vi "HEWH Draw Until.vi"(7 "error in (no error)":errorcluster) -> (0 "error out":errorcluster, 3 "Condition Cluster Output":T4)   [LabVIEW 2019]
uses:
  Utility/Custom Pallet Controls/Custom Pallet DBL.ctl
  Type Definitions/HEWH Power Elements.ctl
  Utility/Custom Pallet Controls/Custom Pallet Forward.ctl
  Utility/Custom Pallet Controls/Custom Pallet Reverse.ctl
  Type Definitions/HEWH Termination Condition Cluster.ctl
panel:
  in  "Mean Tank Temperature Bool":bool
  in  "Mean Tank Temperature":T1 format="%.2f"
  in  "Time":bool
  in  "RTD Temp":bool
  in  "RTD Decrease":bool
  in  "RTD Out Temperature":T1 format="%.2f"
  in  "Time (Seconds)":T1 format="%.2f"
  in  "Return":T2
  in  "Complete":T3
  in  "Decrease RTD Output\nTemperature By\n(Degrees F)":T1 format="%.2f"
  out "Description":string="Draw Until?"
  in  "Tab Control":enum32{"Page 1", "Page 2"}(tab)
  in  "Condition Cluster Input":T4
  in  "Start Draw":bool
  in  "Power Elements":T5
  # "AND/OR"
  # "Select ONLY complete to draw until any heat source"
  # "Select Only One Condition"
  # "Just Draw Water!"
  # "Condition #1"
  # "Draw Until Any Heat Source"
  # "Condition #2"
  # "Start Dispense Pattern"
  # "Draw Until Specific Heat Source"
  # "Condition #3"
  # "Dispense PRAT Sequence"
  # "Not Working"
  # "Condition #4"
  # "Condition #5"
  # "Condition #6"
  # "Select Only One Condition"
  # "Just Draw Water!"
  # "Condition #1"
  # "Draw Until Any Heat Source"
  # "Condition #2"
  # "Start Dispense Pattern"
  # "Draw Until Specific Heat Source"
  # "Condition #3"
  # "Dispense PRAT Sequence"
  # "Not Working"
  # "Condition #4"
  # "Condition #5"
  # "Condition #6"
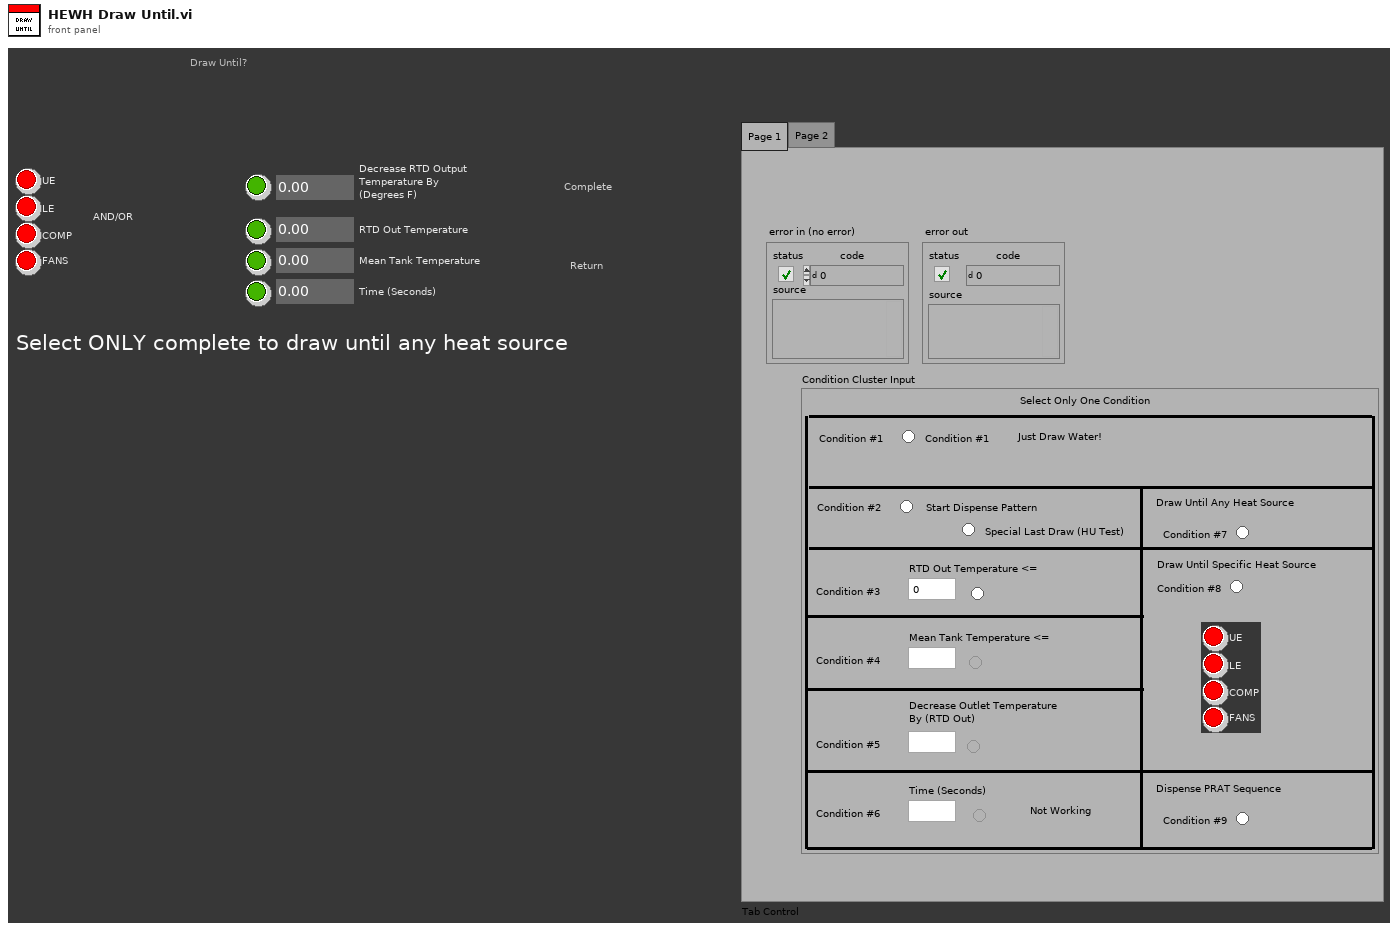
[diagram p1: front panel]
types:
  T1 = typedef "Custom Pallet DBL.ctl" = dbl
  T2 = typedef "Custom Pallet Reverse.ctl" = bool
  T3 = typedef "Custom Pallet Forward.ctl" = bool
  T4 = typedef "HEWH Termination Condition Cluster.ctl" = cluster{"Condition #1":bool, "Condition #2":bool, "Special Last Draw (HU Test)":bool, "RTD Out Temperature <=":dbl, "Condition #3":bool, "Mean Tank Temperature <=":dbl, "Condition #4":bool, "Decrease Outlet Temperature \nBy (RTD Out)":dbl, "Condition #5":bool, "Condition #6":bool, "Time (Seconds)":dbl, "Condition #7":bool, "Condition #8":bool, "Draw Until Condition":T5, "Condition #9":bool}
  T5 = typedef "HEWH Power Elements.ctl" = cluster{"UE":bool, "LE":bool, "COMP":bool, "FANS":bool}
  T6 = enum32{"invalid app kind", "Development System", "Run Time System", "Student Edition", "Embedded LabVIEW", "Evaluation", "Custom"}
  T7 = enum32{"Invalid", "Standard", "Closed", "Hidden", "Minimized", "Maximized"}
  T8 = cluster{"Core":cluster{"Current VI Reference":refnum<vi>, "Close Panel on Exit?":bool}, "Power Elements":T5, "Start Draw":bool, "Decrease RTD Output\nTemperature By\n(Degrees F)":T1, "Return":bool, "Time (Seconds)":T1, "RTD Out Temperature":T1, "Condition Cluster Input":T4, "Mean Tank Temperature":T1}
  T9 = cluster{"Current VI Reference":refnum<vi>, "Close Panel on Exit?":bool}
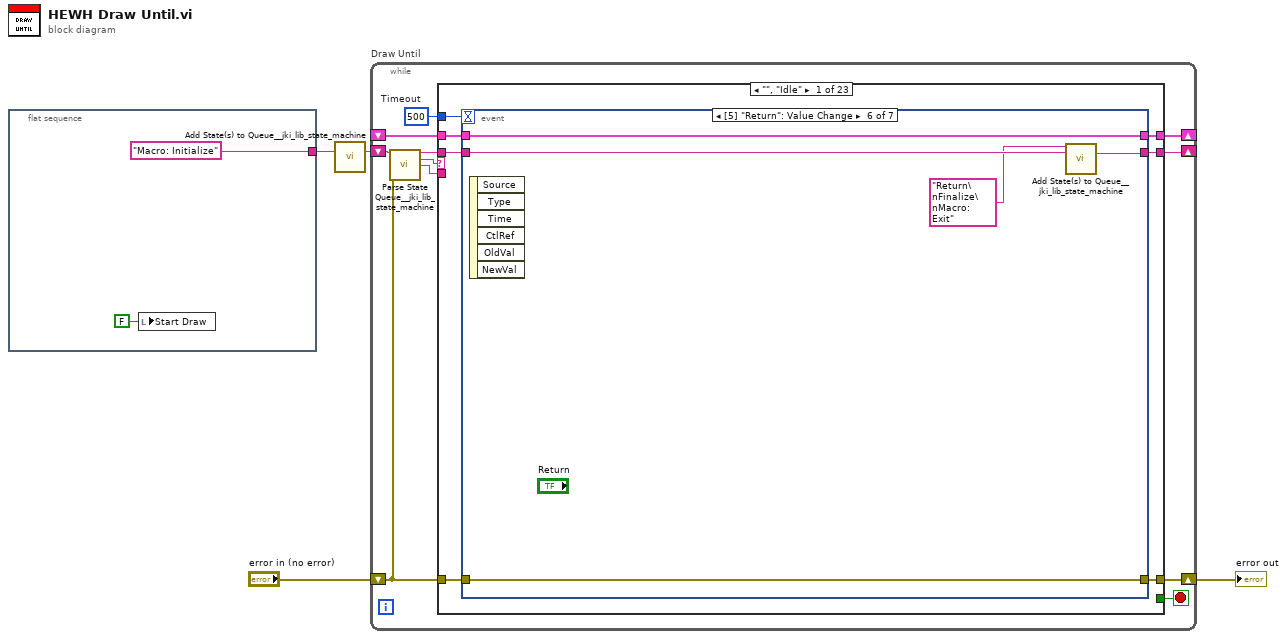
[diagram p0: block diagram]
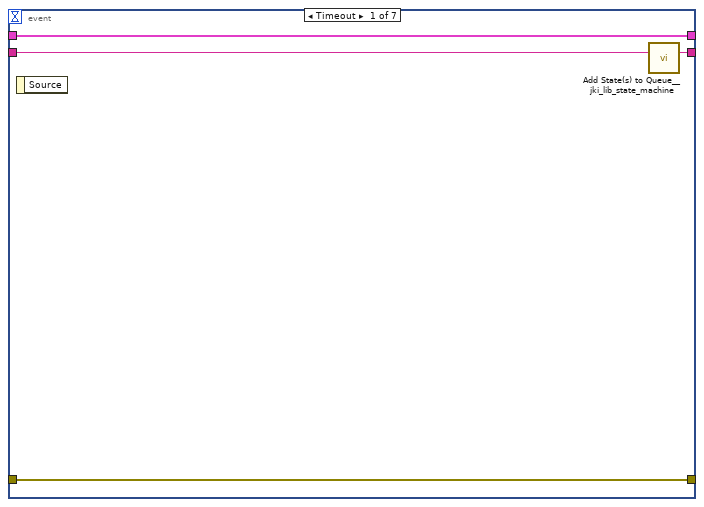
[diagram p2: hidden frame]
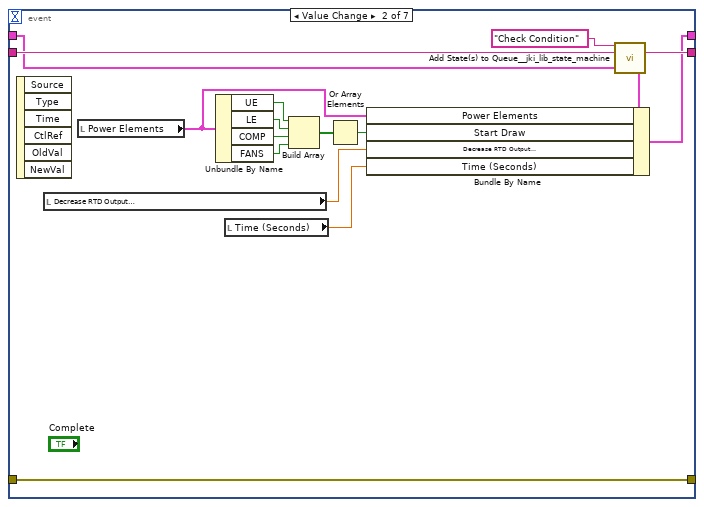
[diagram p3: hidden frame]
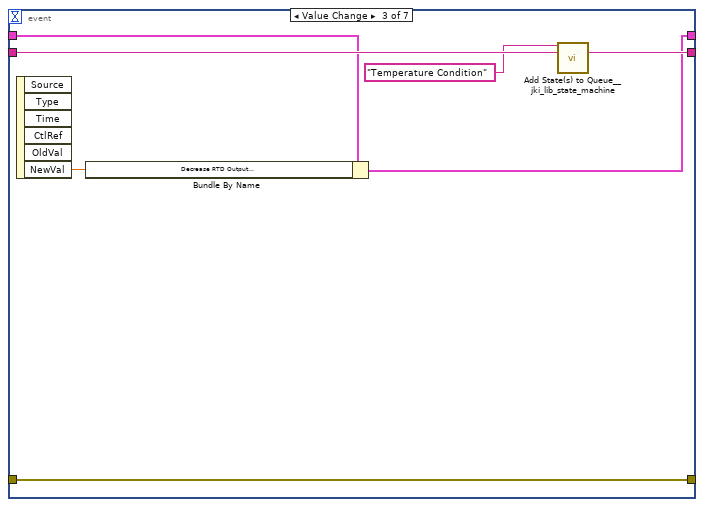
[diagram p4: hidden frame]
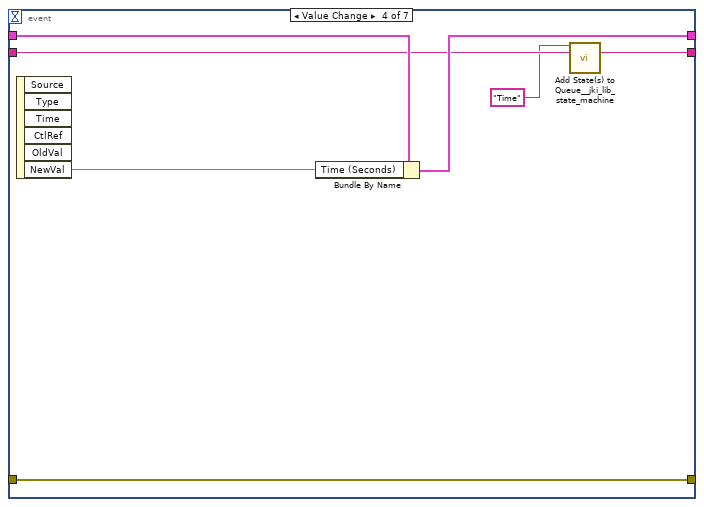
[diagram p5: hidden frame]
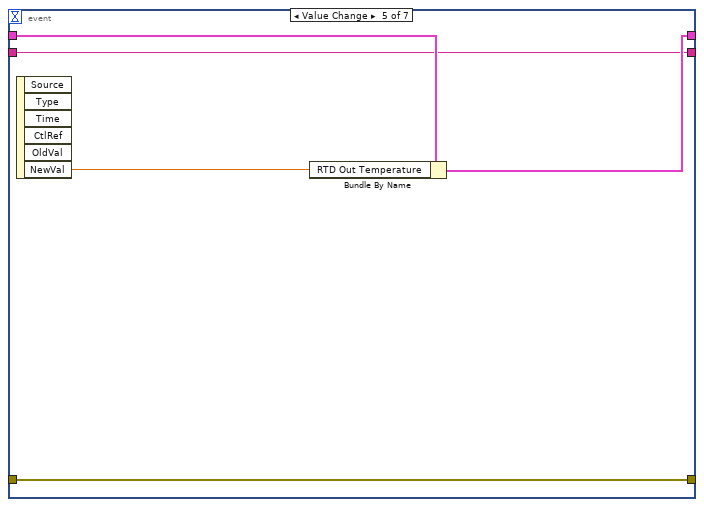
[diagram p6: hidden frame]
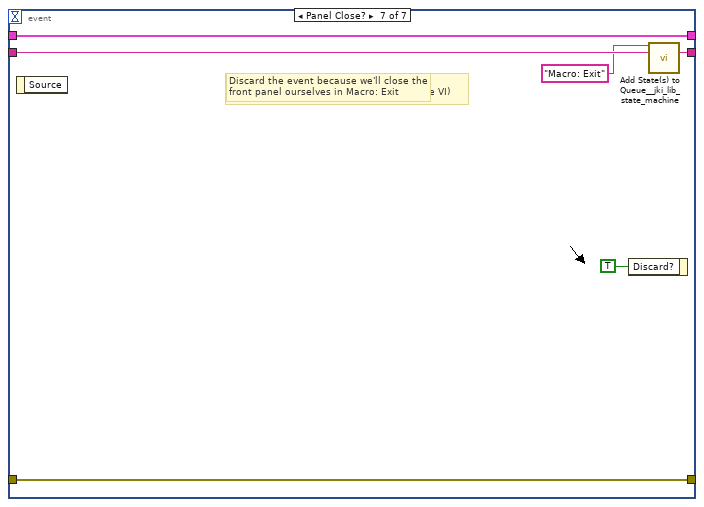
[diagram p7: hidden frame]
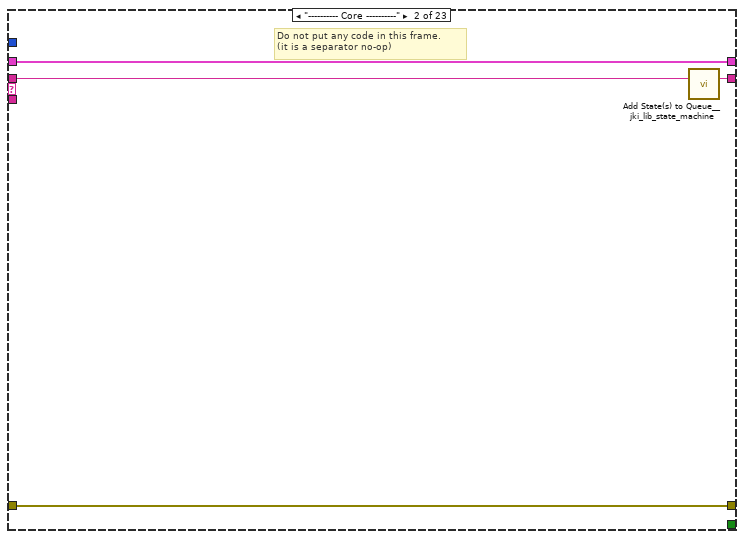
[diagram p8: hidden frame]
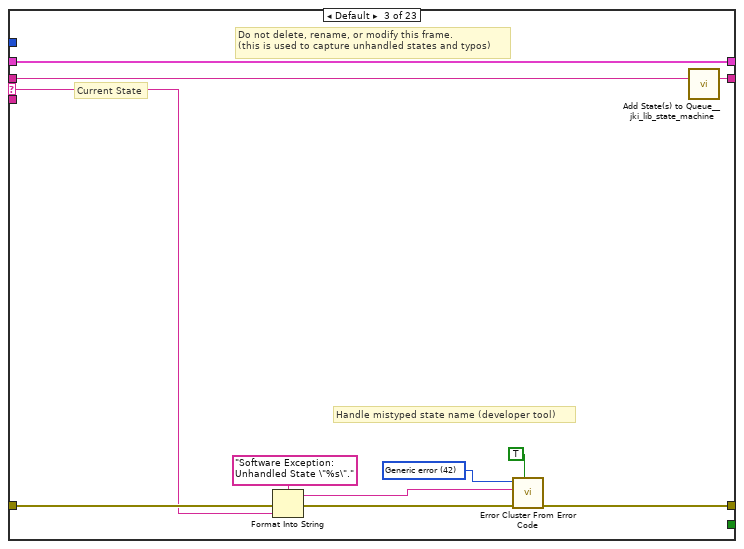
[diagram p9: hidden frame]
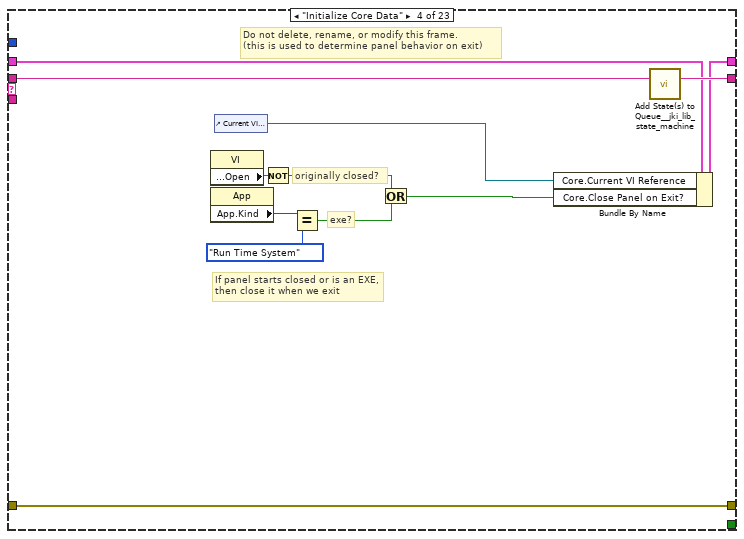
[diagram p10: hidden frame]
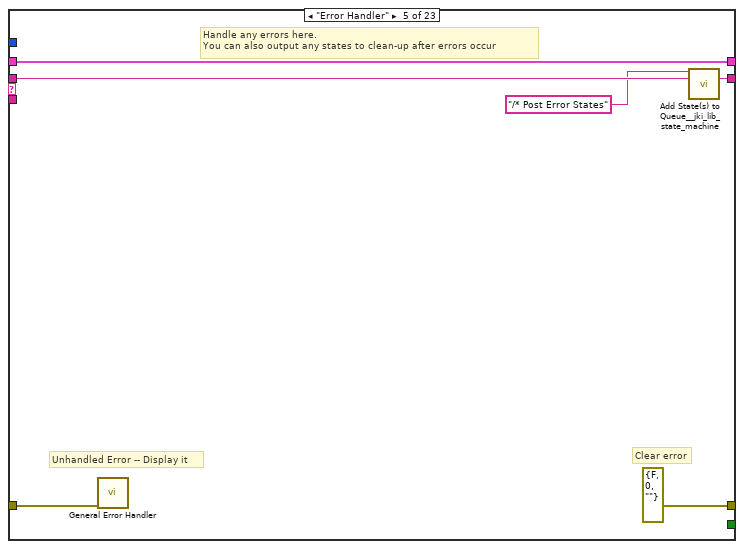
[diagram p11: hidden frame]
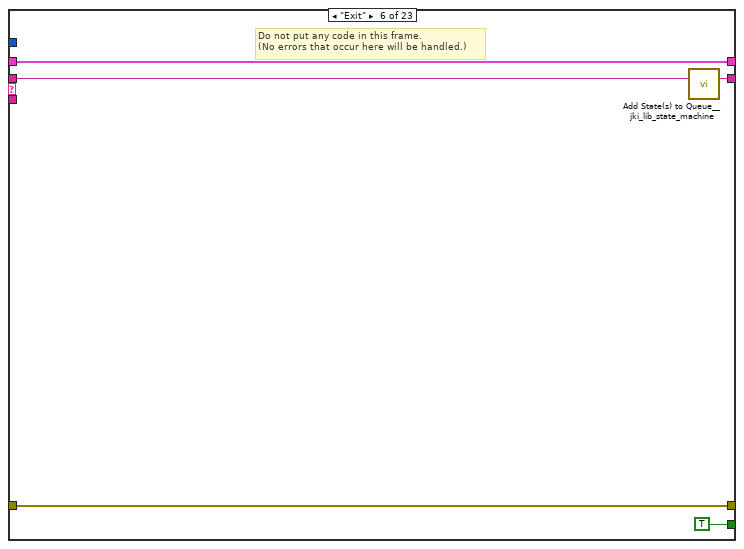
[diagram p12: hidden frame]
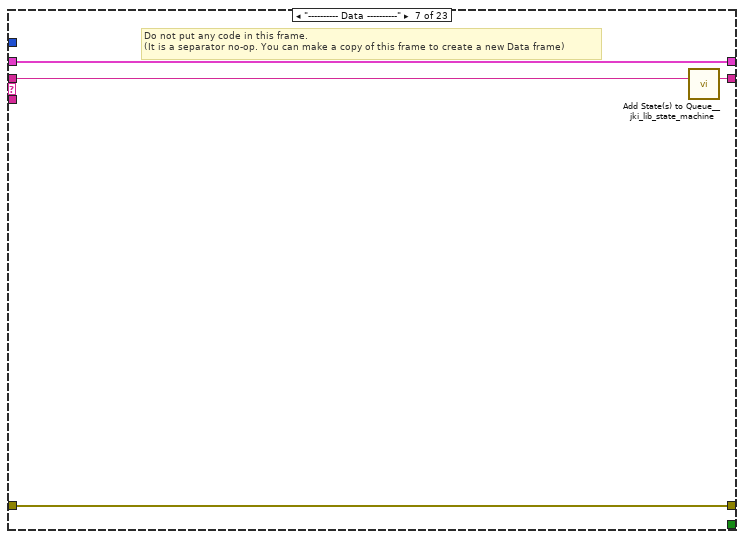
[diagram p13: hidden frame]
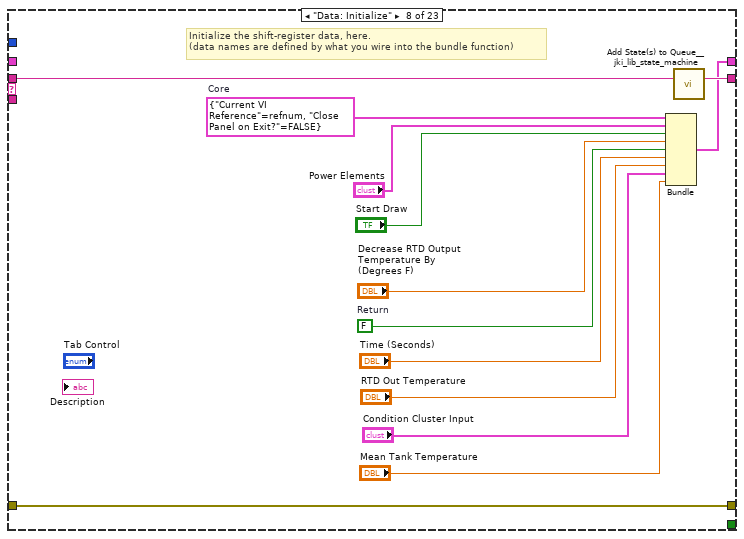
[diagram p14: hidden frame]
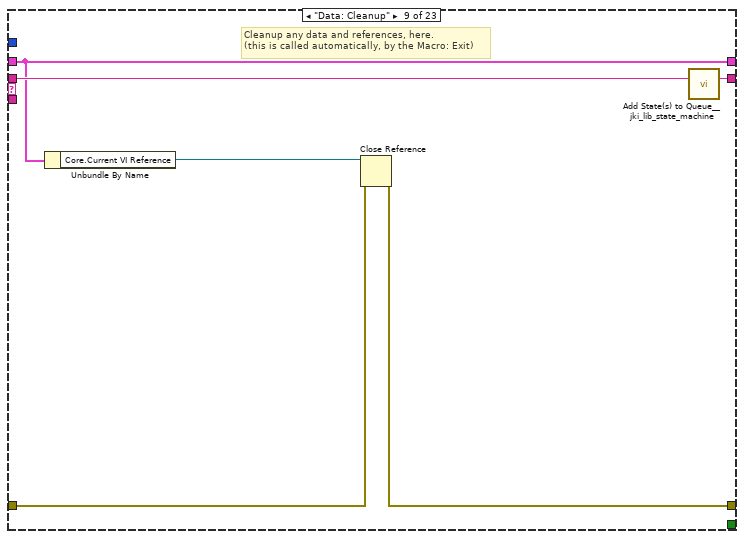
[diagram p15: hidden frame]
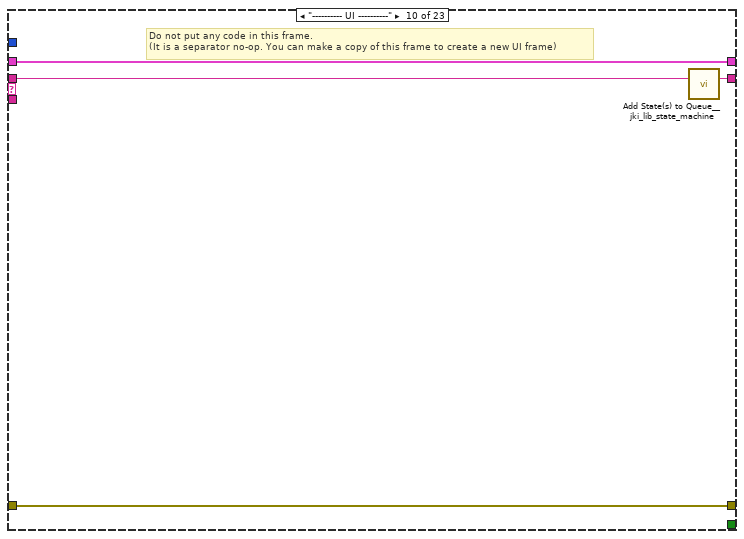
[diagram p16: hidden frame]
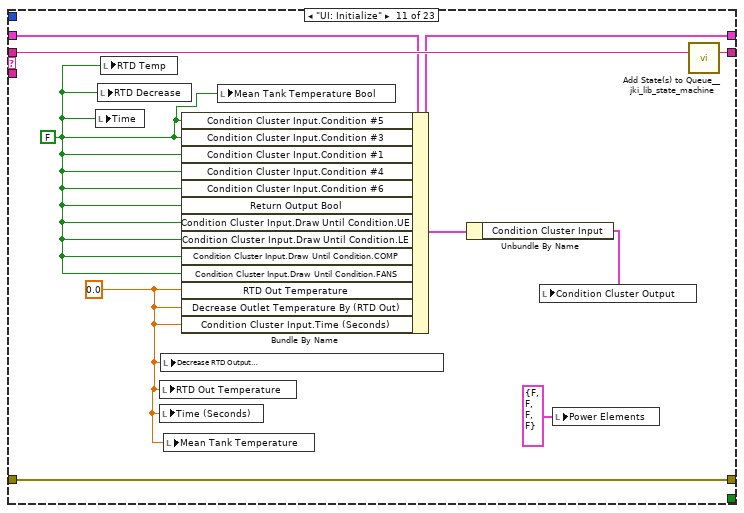
[diagram p17: hidden frame]
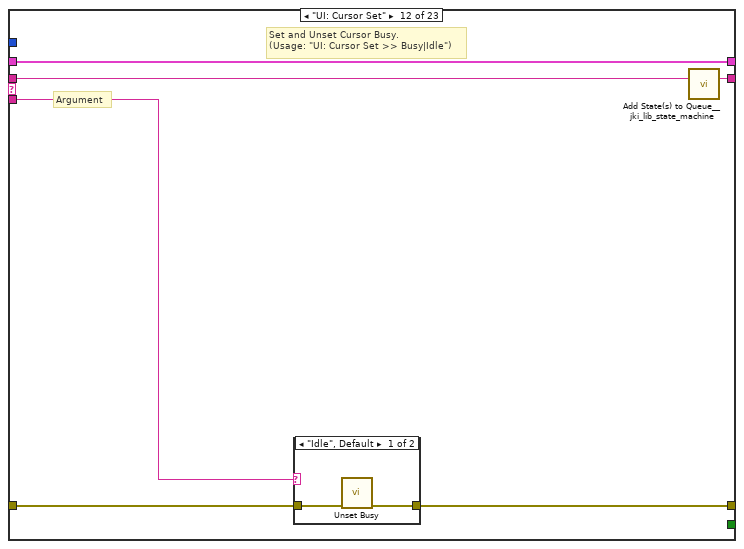
[diagram p18: hidden frame]
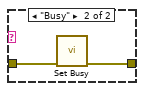
[diagram p19: hidden frame]
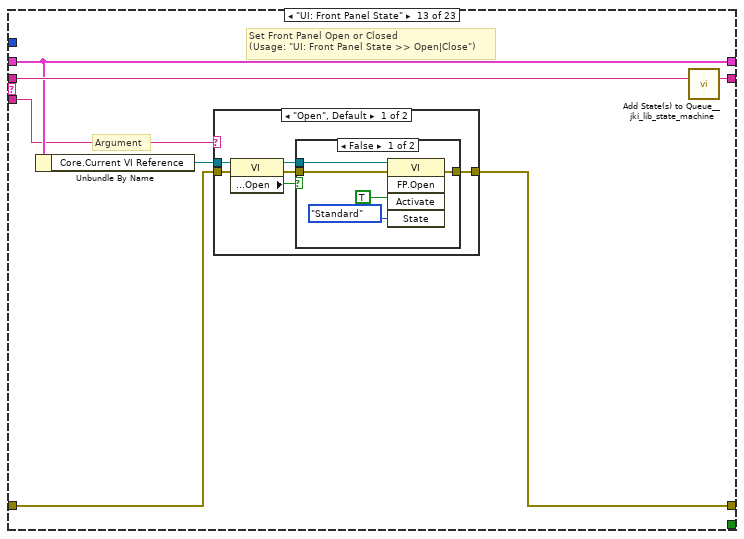
[diagram p20: hidden frame]
diagram:
  n1 = flat-sequence {
    tunnel: ["Macro: Initialize"] -> w3
    frame #0 {
      n2 = local write "Start Draw"(FALSE ("Start Draw")) -> ()
    }
  }
  n3 = call <vilib>:"Add State(s) to Queue__jki_lib_state_machine.vi"("State(s) in (\"\")"=w3) -> ("States Out"=w4:string)  [unwired: 14 in]
  n4 = while "Draw Until" {
    shift-right: [w10] -> _
    shift-left: _ -> [w9]
    shift-right: [w13] -> w2
    shift-left: "error in (no error)" -> [w7]
    shift-right: [w12] -> _
    shift-left: w4 -> [w14]
    stop <- w11 stop-if-true
    w8 = 500  # Timeout
    n5 = call <vilib>:"Parse State Queue__jki_lib_state_machine.vi"("State Queue"=w14, "Error In (no error)"=w7) -> ("Remaining States"=w16:string, "Current State"=w17:string, "Arguments"=w15:string)  [unwired: 11 in]
    n6 = case shown="\"\", \"Idle\"" w17 {
      selector: w17 -> [_ _ w78 _ _ _ _ _ _ _ _ _ _ _ _ _ _ _ _ _ _ _ _]
      tunnel: w16 -> [w24 w77 w82 w100 w106 w111 w115 w128 w134 w138 w147 w153 w164 w190 w195 w205 w209 w235 w255 w261 w265 w271 w276]
      tunnel: w15 -> [_ _ _ _ _ _ _ _ _ _ _ w148 w158 _ _ _ _ _ _ _ _ _ _]
      tunnel: w9 -> [w22 w74 w80 w91 w103 w109 w112 _ w129 w135 w144 w151 w160 w187 w192 w202 w206 w228 w243 w258 w262 w268 w273]
      tunnel: [w21 w75 w84 w97 errorcluster {"status"=FALSE, "code"=0, "source"=""} ("error out") w108 w113 w125 w130 w136 w145 w149 w161 w188 w193 w203 w207 w233 w253 w259 w263 w269 w274] -> w13
      tunnel: w7 -> [w20 w75 w83 w97 w102 w108 w113 w125 w131 w136 w145 w150 w162 w188 w193 w203 w207 w233 w253 w259 w263 w269 w274]
      tunnel: [w23 w76 w81 w99 w105 w110 w114 w127 w133 w137 w146 w152 w163 w189 w194 w204 w208 w234 w254 w260 w264 w270 w275] -> w12
      tunnel: [_ _ _ _ _ TRUE _ _ _ _ _ _ _ _ _ _ _ _ _ _ _ _ _] -> w11
      tunnel: [w18 w74 w80 w98 w103 w109 w112 w126 w129 w135 w143 w151 w160 w187 w192 w202 w206 w227 w242 w257 w262 w267 w273] -> w10
      tunnel: w8 -> [w19 _ _ _ _ _ _ _ _ _ _ _ _ _ _ _ _ _ _ _ _ _ _]
      frame "", "Idle" {
        n7 = event shown="[5] \"Return\": Value Change" {
          selector: _ -> [_ _ _ _ _ _ _]
          dyn-events: _ -> [_ _ _ _ _ _ _]
          timeout: w19 -> [_ _ _ _ _ _ _]
          tunnel: w24 -> [w28 w42 w49 w53 w58 w64 w73]
          tunnel: [w27 w43 w48 w52 w58 w65 w72] -> w23
          tunnel: w22 -> [w25 w40 w46 w56 w61 w66 w70]
          tunnel: [w26 w41 w50 w57 w62 w67 w71] -> w21
          tunnel: w20 -> [w26 w41 w50 w57 w62 w67 w71]
          tunnel: [w25 w39 w45 w55 w60 w66 w70] -> w18
          event Timeout {
            n8 = event-data() -> ()  [unwired: 1 in, 1 out]
            n9 = call <vilib>:"Add State(s) to Queue__jki_lib_state_machine.vi"("State(s) in (\"\")"=w28) -> ("States Out"=w27:string)  [unwired: 14 in]
          }
          event Value Change {
            n10 = event-data() -> ()  [unwired: 1 in, 6 out]
            n11 = local read "Decrease RTD Output\nTemperature By\n(Degrees F)"() -> (w38:T1)
            n12 = local read "Power Elements"() -> (w29:T5)
            n13 = Unbundle By Name(w29) -> ("UE"=w35:bool, "LE"=w34:bool, "COMP"=w33:bool, "FANS"=w32:bool)
            n14 = local read "Time (Seconds)"() -> (w37:T1)
            n15 = Build Array(w35, w34, w33, w32) -> (w31:bool[])
            n16 = Or Array Elements(Boolean array=w31) -> (logical OR=w30:bool)
            n17 = Bundle By Name(cluster=w40, "Power Elements"=w29, "Start Draw"=w30, "Decrease RTD Output\nTemperature By\n(Degrees F)"=w38, "Time (Seconds)"=w37) -> (w39:T8)
            n18 = call <vilib>:"Add State(s) to Queue__jki_lib_state_machine.vi"("State(s) in Front (\"\")"="Check Condition" ("State(s) in Front (\"\")"), "State(s) in (\"\")"=w42) -> ("States Out"=w43:string)  [unwired: 13 in]
          }
          event Value Change {
            n19 = event-data() -> ("NewVal"=w44:T1)  [unwired: 1 in, 5 out]
            n20 = Bundle By Name(cluster=w46, "Decrease RTD Output\nTemperature By\n(Degrees F)"=w44) -> (w45:T8)
            n21 = call <vilib>:"Add State(s) to Queue__jki_lib_state_machine.vi"("State(s) in Front (\"\")"="Temperature Condition" ("State(s) in Front (\"\")"), "State(s) in (\"\")"=w49) -> ("States Out"=w48:string)  [unwired: 13 in]
          }
          event Value Change {
            n22 = event-data() -> ("NewVal"=w54:T1)  [unwired: 1 in, 5 out]
            n23 = Bundle By Name(cluster=w56, "Time (Seconds)"=w54) -> (w55:T8)
            n24 = call <vilib>:"Add State(s) to Queue__jki_lib_state_machine.vi"("State(s) in Front (\"\")"="Time" ("State(s) in Front (\"\")"), "State(s) in (\"\")"=w53) -> ("States Out"=w52:string)  [unwired: 13 in]
          }
          event Value Change {
            n25 = event-data() -> ("NewVal"=w59:T1)  [unwired: 1 in, 5 out]
            n26 = Bundle By Name(cluster=w61, "RTD Out Temperature"=w59) -> (w60:T8)
          }
          event Value Change {
            n27 = event-data() -> ()  [unwired: 1 in, 6 out]
            n28 = call <vilib>:"Add State(s) to Queue__jki_lib_state_machine.vi"("State(s) in Front (\"\")"="Return\nFinalize\nMacro: Exit", "State(s) in (\"\")"=w64) -> ("States Out"=w65:string)  [unwired: 13 in]
          }
          event Panel Close? {
            # "Discard the event because we'll close the front panel ourselves in Macro: Exit"
            # "Close Panel button (pressed) Event\n(this executes Macro: Exit to terminate the VI)"
            n29 = event-data() -> ()  [unwired: 1 in, 1 out]
            n30 = event-data("Discard?"=TRUE) -> ()  [unwired: 1 in, 1 out]
            n31 = call <vilib>:"Add State(s) to Queue__jki_lib_state_machine.vi"("State(s) in Front (\"\")"="Macro: Exit", "State(s) in (\"\")"=w73) -> ("States Out"=w72:string)  [unwired: 13 in]
          }
        }
      }
      frame "---------- Core ----------" {
        # "Do not put any code in this frame.\n(it is a separator no-op)"
        n32 = call <vilib>:"Add State(s) to Queue__jki_lib_state_machine.vi"("State(s) in (\"\")"=w77) -> ("States Out"=w76:string)  [unwired: 14 in]
      }
      frame Default {
        w87 = 42 items=["No error", "Argument error", "Memory is full", "Out of zone", "End of file", "File already open", "Generic file I/O error", "File not found", "File permission error", "Disk is full", "Duplicate path", "Too many files open", "System feature not enabled", "Resource file not found", "Cannot add resource", "Resource not found", "Image not found", "Image memory error", "Pen does not exist", "Config type invalid", "Config token not found", "Config parse error", "Config memory error", "Bad external code format", "Bad external code offset", "External code not present", "Null window", "Destroy window error", "Null menu", "Print aborted", "Bad print record", "Print driver error", "Windows error during printing", "Memory error during printing", "Print dialog error", "Generic print error", "Invalid device refnum", "Device not found", "Device parameter error", "Device unit error", "Cannot open device", "Device call aborted", "Generic error", "Cancelled by user", "Object ID too low", "Object ID too high", "Object not in heap", "Unknown heap", "Unknown object (invalid DefProc)", "Unknown object (DefProc not in table)", "Message out of range", "Invalid (null) method", "Unknown message", "Manager call not supported", "Bad address", "Network operation in progress", "Network operation timed out", "Connection is busy", "Network attribute not supported", "Network error", "Address in use", "System out of memory", "Connection aborted", "Connection refused", "Not connected", "Already connected", "Connection closed", "Initialization error (interapplication manager)", "Bad occurrence", "Wait on unbound occurrence handler", "Occurrence queue overflow", "Datalog type conflict", "Unused", "Unrecognized type (interapplication manager)", "Memory corrupt", "Failed to make temporary DLL", "Old CIN version", "Drag socket not found", "Failed to load drop-object", "Failed to register OLE object", "Failed to release OLE object", "Format specifier type mismatch", "Unknown format specifier", "Too few format specifiers", "Too many format specifiers", "Scan failed", "Newer CIN version", "Error converting to variant", "Runtime menu error", "Password tampered", "Variant attribute not found", "Incompatible variant data type", "Event data is not available", "Event Store is not present", "Occurrence is not found", "Event Queue is not created", "Event info is not available", "Refnum passed is NULL", "Error retrieving Class GUID", "Error retrieving CoClass GUID", "Error retrieving TypeLib GUID.", "Bad built application magic bytes.", "Specific driver is different from the specific driver associated with the Logical Name.", "There is no session opened to the class driver.", "Max Error", "MAX - Error with config objects", "MAX - Error loading configuration", "MAX - Group not supported"]
        # "Current State"
        # "Do not delete, rename, or modify this frame.\n(this is used to capture unhandled states and typos)"
        # "Handle mistyped state name (developer tool)"
        n33 = Format Into String(format string="Software Exception: Unhandled State \"%s\"." ("message"), error in=w83, w78) -> (resulting string=w86:string, error out=w85:errorcluster)  [unwired: 1 in]
        n34 = call <vilib>:"Error Cluster From Error Code.vi"("show call chain? (False)"=TRUE, "error in (no error)"=w85, "error message (\"\")"=w86, "error code (0)"=w87) -> ("error out"=w84:errorcluster)  [unwired: 5 in]
        n35 = call <vilib>:"Add State(s) to Queue__jki_lib_state_machine.vi"("State(s) in (\"\")"=w82) -> ("States Out"=w81:string)  [unwired: 14 in]
      }
      frame "Initialize Core Data" {
        # "Do not delete, rename, or modify this frame.\n(this is used to determine panel behavior on exit)"
        # "originally closed?"
        # "exe?"
        # "If panel starts closed or is an EXE, then close it when we exit"
        n36 = property class="VI"() -> ("Front Panel.Open"=w96:bool)  [unwired: 2 in, 2 out]
        n37 = property class="App"() -> ("App.Kind"=w95:T6)  [unwired: 2 in, 2 out]
        n38 = control-ref of="Current VI Reference"() -> (w89:refnum<vi>)
        n39 = Not(x=w96) -> (.not. x?=w93:bool)
        n40 = Equal?(x=w95, y=T6."Run Time System" ("Application:Kind")) -> (x = y?=w92:bool)
        n41 = Or(x=w93, y=w92) -> (x .or. y?=w90:bool)
        n42 = Bundle By Name(cluster=w91, "Core.Current VI Reference"=w89, "Core.Close Panel on Exit?"=w90) -> (w98:T8)
        n43 = call <vilib>:"Add State(s) to Queue__jki_lib_state_machine.vi"("State(s) in (\"\")"=w100) -> ("States Out"=w99:string)  [unwired: 14 in]
      }
      frame "Error Handler" {
        # "Unhandled Error -- Display it"
        # "Handle any errors here.\nYou can also output any states to clean-up after errors occur"
        # "Clear error"
        n44 = call <vilib>:"General Error Handler.vi"("error in (no error)"=w102) -> ()  [unwired: 10 in, 5 out]
        n45 = call <vilib>:"Add State(s) to Queue__jki_lib_state_machine.vi"("State(s) in Front (\"\")"="/* Post Error States", "State(s) in (\"\")"=w106) -> ("States Out"=w105:string)  [unwired: 13 in]
      }
      frame "Exit" {
        # "Do not put any code in this frame.\n(No errors that occur here will be handled.)"
        n46 = call <vilib>:"Add State(s) to Queue__jki_lib_state_machine.vi"("State(s) in (\"\")"=w111) -> ("States Out"=w110:string)  [unwired: 14 in]
      }
      frame "---------- Data ----------" {
        # "Do not put any code in this frame.\n(It is a separator no-op. You can make a copy of this frame to create a new Data frame)"
        n47 = call <vilib>:"Add State(s) to Queue__jki_lib_state_machine.vi"("State(s) in (\"\")"=w115) -> ("States Out"=w114:string)  [unwired: 14 in]
      }
      frame "Data: Initialize" {
        w120 = FALSE  # Return
        w124 = T9 {"Current VI Reference"=refnum, "Close Panel on Exit?"=FALSE}  # Core
        # "Initialize the shift-register data, here.\n(data names are defined by what you wire into the bundle function)"
        n48 = Bundle("Core"=w124, "Power Elements"="Power Elements", "Start Draw"="Start Draw", "Decrease RTD Output\nTemperature By\n(Degrees F)"="Decrease RTD Output\nTemperature By\n(Degrees F)", "Return"=w120, "Time (Seconds)"="Time (Seconds)", "RTD Out Temperature"="RTD Out Temperature", "Condition Cluster Input"="Condition Cluster Input", "Mean Tank Temperature"="Mean Tank Temperature") -> (w126:T8)  [unwired: 1 in]
        n49 = call <vilib>:"Add State(s) to Queue__jki_lib_state_machine.vi"("State(s) in (\"\")"=w128) -> ("States Out"=w127:string)  [unwired: 14 in]
      }
      frame "Data: Cleanup" {
        # "Cleanup any data and references, here.\n(this is called automatically, by the Macro: Exit)"
        n50 = Unbundle By Name(w129) -> ("Core.Current VI Reference"=w132:refnum<vi>)
        n51 = Close Reference(reference=w132, error in (no error)=w131) -> (error out=w130:errorcluster)
        n52 = call <vilib>:"Add State(s) to Queue__jki_lib_state_machine.vi"("State(s) in (\"\")"=w134) -> ("States Out"=w133:string)  [unwired: 14 in]
      }
      frame "---------- UI ----------" {
        # "Do not put any code in this frame.\n(It is a separator no-op. You can make a copy of this frame to create a new UI frame)"
        n53 = call <vilib>:"Add State(s) to Queue__jki_lib_state_machine.vi"("State(s) in (\"\")"=w138) -> ("States Out"=w137:string)  [unwired: 14 in]
      }
      frame "UI: Initialize" {
        w139 = T1 0.0 ("Condition Cluster Input.RTD Out Temperature Output")
        w140 = FALSE ("Condition Cluster Input.Decrease RTD Output\nTemperature By\n(Degrees F)")
        n54 = local write "Time"(w140) -> ()
        n55 = local write "RTD Decrease"(w140) -> ()
        n56 = local write "RTD Temp"(w140) -> ()
        n57 = local write "RTD Out Temperature"(w139) -> ()
        n58 = local write "Time (Seconds)"(w139) -> ()
        n59 = local write "Decrease RTD Output\nTemperature By\n(Degrees F)"(w139) -> ()
        n60 = local write "Mean Tank Temperature"(w139) -> ()
        n61 = Bundle By Name(cluster=w144, "Condition Cluster Input.Condition #5"=w140, "Condition Cluster Input.Condition #3"=w140, "Condition Cluster Input.Condition #1"=w140, "Condition Cluster Input.Condition #4"=w140, "Condition Cluster Input.Condition #6"=w140, "Return Output Bool"=w140, "Condition Cluster Input.Draw Until Condition.UE"=w140, "Condition Cluster Input.Draw Until Condition.LE"=w140, "Condition Cluster Input.Draw Until Condition.COMP"=w140, "Condition Cluster Input.Draw Until Condition.FANS"=w140, "RTD Out Temperature"=w139, "Decrease Outlet Temperature By (RTD Out)"=w139, "Condition Cluster Input.Time (Seconds)"=w139) -> (w143:T8)
        n62 = local write "Mean Tank Temperature Bool"(w140) -> ()
        n63 = Unbundle By Name(w143) -> ("Condition Cluster Input"=w142:T4)
        n64 = local write "Condition Cluster Output"(w142) -> ()
        n65 = local write "Power Elements"(T5 {"UE"=FALSE, "LE"=FALSE, "COMP"=FALSE, "FANS"=FALSE} ("Power Elements")) -> ()
        n66 = call <vilib>:"Add State(s) to Queue__jki_lib_state_machine.vi"("State(s) in (\"\")"=w147) -> ("States Out"=w146:string)  [unwired: 14 in]
      }
      frame "UI: Cursor Set" {
        # "Argument"
        # "Set and Unset Cursor Busy.\n(Usage: \"UI: Cursor Set >> Busy|Idle\")"
        n67 = case shown="\"Idle\", Default" w148 {
          tunnel: w150 -> [w155 w157]
          tunnel: [w154 w156] -> w149
          frame "Idle", Default {
            n68 = call <vilib>:"Unset Busy.vi"("error in (no error)"=w155) -> ("error out"=w154:errorcluster)  [unwired: 10 in]
          }
          frame "Busy" {
            n69 = call <vilib>:"Set Busy.vi"("error in (no error)"=w157) -> ("error out"=w156:errorcluster)  [unwired: 9 in, 1 out]
          }
        }
        n70 = call <vilib>:"Add State(s) to Queue__jki_lib_state_machine.vi"("State(s) in (\"\")"=w153) -> ("States Out"=w152:string)  [unwired: 14 in]
      }
      frame "UI: Front Panel State" {
        # "Argument"
        # "Set Front Panel Open or Closed\n(Usage: \"UI: Front Panel State >> Open|Close\")"
        n71 = Unbundle By Name(w160) -> ("Core.Current VI Reference"=w159:refnum<vi>)
        n72 = case shown="\"Open\", Default" w158 {
          tunnel: w162 -> [w168 w181]
          tunnel: [w170 w182] -> w161
          tunnel: w159 -> [w169 w179]
          frame "Open", Default {
            n73 = property class="VI"(reference=w169, error in=w168) -> (reference out=w166:refnum<vi>, error out=w167:errorcluster, "Front Panel.Open"=w165:bool)
            n74 = case shown="False" w165 {
              tunnel: [w173 w176] -> w170
              tunnel: w167 -> [w172 w176]
              tunnel: w166 -> [w171 _]
              frame False {
                n75 = invoke class="VI" method="FP.Open"(reference=w171, error in=w172, "Activate"=TRUE, "State"=T7."Standard") -> (error out=w173:errorcluster)  [unwired: 1 in, 4 out]
              }
              frame True {
              }
            }
          }
          frame "Close" {
            n76 = property class="VI"(reference=w179, error in=w181) -> (reference out=w178:refnum<vi>, error out=w180:errorcluster, "Front Panel.Open"=w177:bool)
            n77 = case shown="True" w177 {
              tunnel: [w183 w186] -> w182
              tunnel: w180 -> [w183 w185]
              tunnel: w178 -> [_ w184]
              frame False {
              }
              frame True {
                n78 = invoke class="VI" method="FP.Close"(reference=w184, error in=w185) -> (error out=w186:errorcluster)  [unwired: 1 in, 2 out]
              }
            }
          }
        }
        n79 = call <vilib>:"Add State(s) to Queue__jki_lib_state_machine.vi"("State(s) in (\"\")"=w164) -> ("States Out"=w163:string)  [unwired: 14 in]
      }
      frame "---------- Macro ----------" {
        # "Do not put any code in this frame.\n(It is a separator no-op. You can make a copy of this frame to create a new Macro frame)"
        n80 = call <vilib>:"Add State(s) to Queue__jki_lib_state_machine.vi"("State(s) in (\"\")"=w190) -> ("States Out"=w189:string)  [unwired: 14 in]
      }
      frame "Macro: Initialize" {
        w191 = "Data: Initialize\nInitialize Core Data\nUI: Initialize\nUI: Front Panel State >> Open"  # Data: Initialize Initialize Core Data UI: Initialize UI: Front Panel State >> Open
        # "Initialization Macro\n(This is called once, when the VI starts)"
        n81 = call <vilib>:"Add State(s) to Queue__jki_lib_state_machine.vi"("State(s) in Front (\"\")"=w191, "State(s) in (\"\")"=w195) -> ("States Out"=w194:string)  [unwired: 13 in]
      }
      frame "Macro: Exit" {
        # "Exit Macro\n(This is called once, when the VI exits)"
        n82 = Unbundle By Name(w202) -> ("Core.Close Panel on Exit?"=w201:bool)
        n83 = Select(t="UI: Front Panel State >> Close", s=w201, f="") -> (s? t:f=w198:string)
        n84 = call <vilib>:"Add State(s) to Queue__jki_lib_state_machine.vi"("State(s) in (\"\")"=w198, "State(s) at Back (\"\")"="Data: Cleanup\nExit") -> ("States Out"=w196:string)  [unwired: 13 in]
        n85 = call <vilib>:"Add State(s) to Queue__jki_lib_state_machine.vi"("State(s) in Front (\"\")"=w196, "State(s) in (\"\")"=w205) -> ("States Out"=w204:string)  [unwired: 13 in]
      }
      frame "---------- New Category ----------" {
        # "Template Separator\n(You can make a copy of, or modify, this frame)"
        n86 = call <vilib>:"Add State(s) to Queue__jki_lib_state_machine.vi"("State(s) in (\"\")"=w209) -> ("States Out"=w208:string)  [unwired: 14 in]
      }
      frame "Check Condition" {
        n87 = Unbundle By Name(w228) -> ("Power Elements.UE"=w226:bool, "Power Elements.LE"=w225:bool, "Power Elements.COMP"=w224:bool, "Power Elements.FANS"=w223:bool)
        n88 = local read "Mean Tank Temperature Bool"() -> (w217:bool)
        n89 = local read "Time"() -> (w231:bool)
        n90 = Build Array(w226, w225, w224, w223) -> (w221:bool[])
        n91 = Build Array(w217, "RTD Decrease", "RTD Temp", w231) -> (w230:bool[])
        n92 = Build Array(w217, "RTD Decrease", "RTD Temp") -> (w214:bool[])
        n93 = Or Array Elements(Boolean array=w221) -> (logical OR=w222:bool)
        n94 = Or Array Elements(Boolean array=w230) -> (logical OR=w229:bool)
        n95 = Boolean To (0,1)(Boolean=w214) -> (0, 1=w213:i16[])
        n96 = Not(x=w222) -> (.not. x?=w219:bool)
        n97 = Not(x=w229) -> (.not. x?=w220:bool)
        n98 = Add Array Elements(numeric array=w213) -> (sum=w212:i16)
        n99 = And(x=w220, y=w219) -> (x .and. y?=w218:bool)
        n100 = Greater?(x=w212, y=i16 1) -> (0:w210:bool)
        n101 = case shown="True" w210 {
          tunnel: ["Draw Until Condition\nFinalize\nMacro: Exit" ("State(s) in Front (\"\")") ""] -> w232
          frame False {
          }
          frame True {
            n102 = One Button Dialog(message="Select Only ONE \nTemperature Condition") -> ()  [unwired: 1 in, 1 out]
          }
        }
        n103 = Bundle By Name(cluster=w228, "Condition Cluster Input.Condition #5"=w218) -> (w227:T8)
        n104 = call <vilib>:"Add State(s) to Queue__jki_lib_state_machine.vi"("State(s) in Front (\"\")"=w232, "State(s) in (\"\")"=w235) -> ("States Out"=w234:string)  [unwired: 13 in]
      }
      frame "Draw Until Condition" {
        n105 = Unbundle By Name(w243) -> ("Condition Cluster Input"=w244:T4, "Start Draw"=w245:bool, "Power Elements"=w246:T5, "Decrease RTD Output\nTemperature By\n(Degrees F)"=w249:T1, "Time (Seconds)"=w248:T1, "RTD Out Temperature"=w247:T1)
        n106 = local read "RTD Decrease"() -> (w252:bool)
        n107 = local read "RTD Temp"() -> (w251:bool)
        n108 = local read "Mean Tank Temperature"() -> (w239:T1)
        n109 = Bundle By Name(cluster=w244, "Condition #6"=w245, "Draw Until Condition"=w246, "Decrease Outlet Temperature By (RTD Out)"=w249, "Time (Seconds)"=w248, "RTD Out Temperature"=w247, "Condition #3"=w252, "Condition #1"=w251, "Condition #4"="Time", "Condition #2"="Mean Tank Temperature Bool", "Mean Tank Temperature"=w239) -> (w241:T4)
        n110 = Bundle By Name(cluster=w243, "Condition Cluster Input"=w241) -> (w242:T8)
        n111 = call <vilib>:"Add State(s) to Queue__jki_lib_state_machine.vi"("State(s) in (\"\")"=w255) -> ("States Out"=w254:string)  [unwired: 14 in]
      }
      frame "Temperature Condition" {
        n112 = Bundle By Name(cluster=w258, "Return"=TRUE ("Use Temperature Condition")) -> (w257:T8)
        n113 = call <vilib>:"Add State(s) to Queue__jki_lib_state_machine.vi"("State(s) in (\"\")"=w261) -> ("States Out"=w260:string)  [unwired: 14 in]
      }
      frame "Time" {
        n114 = call <vilib>:"Add State(s) to Queue__jki_lib_state_machine.vi"("State(s) in (\"\")"=w265) -> ("States Out"=w264:string)  [unwired: 14 in]
      }
      frame "Return" {
        n115 = Bundle By Name(cluster=w268, "Return Output Bool"=TRUE ("Condition Cluster Input.Return Output")) -> (w267:T8)
        n116 = call <vilib>:"Add State(s) to Queue__jki_lib_state_machine.vi"("State(s) in (\"\")"=w271) -> ("States Out"=w270:string)  [unwired: 14 in]
      }
      frame "Finalize" {
        n117 = Unbundle By Name(w273) -> ("Condition Cluster Input"=→"Condition Cluster Output":T4)
        n118 = call <vilib>:"Add State(s) to Queue__jki_lib_state_machine.vi"("State(s) in (\"\")"=w276) -> ("States Out"=w275:string)  [unwired: 14 in]
      }
    }
  }
  "error out" <- w2
